vi "CPP-5168-PressureAnalysis.vi"() -> (5 "Plug in titles":string[](array[string]), 7 "Plug in values":string[](array[string]))   [LabVIEW 2011]
uses:
  Globals/Plug_in_data_global.vi
  Globals/Meas_global.vi
panel:
  out "ZeroedCompensatedCalibratedData":dbl[][](array[numeric])
  out "ChannelNames":string[](array[string])
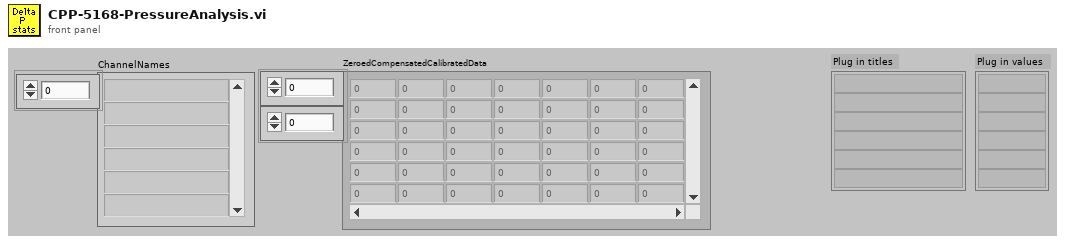
[diagram p1: front panel]
types:
  T1 = typedef "Analysis_info_cluster.ctl" = cluster{"Colour":u32, "Inst type":T2, "Inst name":string, "Symbol":string, "Code name":string, "Extra Info":string, "Inst Array":T3, "Index":i32, "Voltage Index":i32, "Extra Titles":string[], "Extra Values":string[]}
  T2 = typedef "Inst_type.ctl" = enum16{"Propeller anemometer", "Raw voltage", "Pressure Transducer", "Pitot-static tube", "Preston tube", "Hot wire", "Cross wire 1", "Cross wire 2", "Generic Linear", "Generic Polynomial", "Generic BackPoly", "Fast FID", "Thermocouple", "Cold wire", "Pulsed Wire", "LDA Vel", "LDA Tran time", "LDA Arr time"}
  T3 = typedef "Instrument_Array.ctl" = enum16{"PWA", "LDA", "Analogue"}
  T4 = typedef "WindowDescriptor.ctl" = cluster{"WindowName":string, "SurroundingTaps":string[], "TapWeights":dbl[], "OpenAreaFraction":dbl}
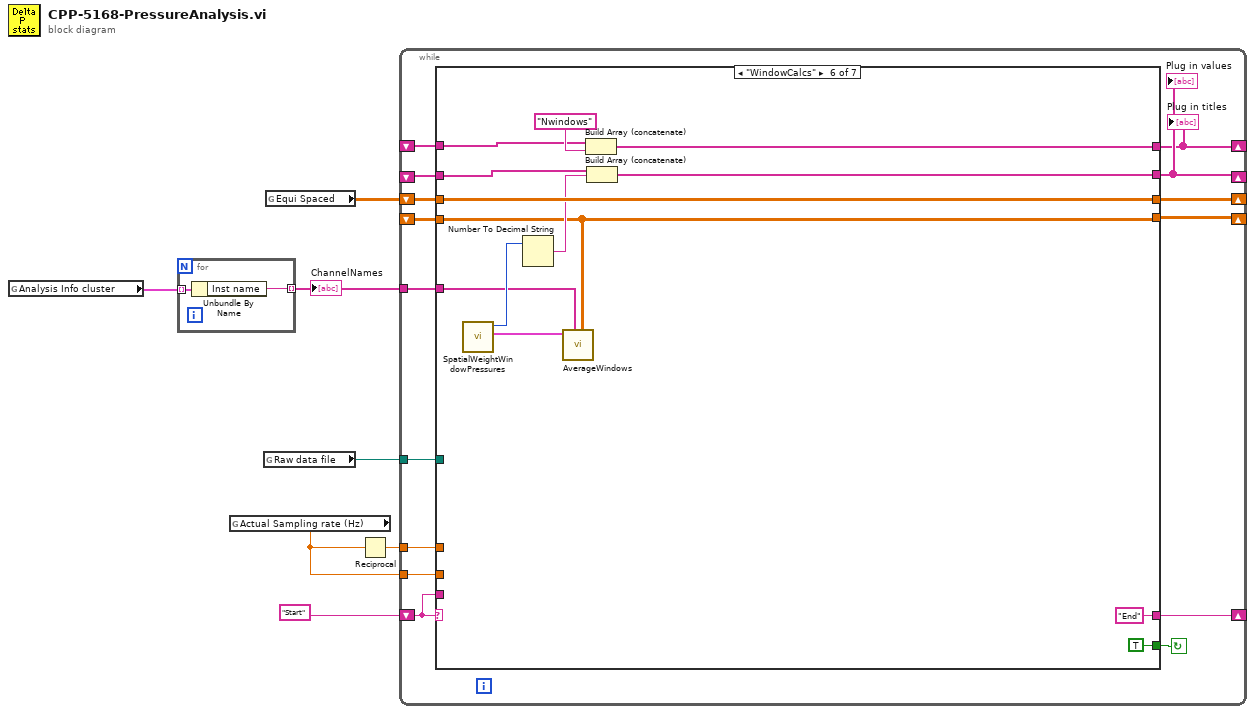
[diagram p0: block diagram]
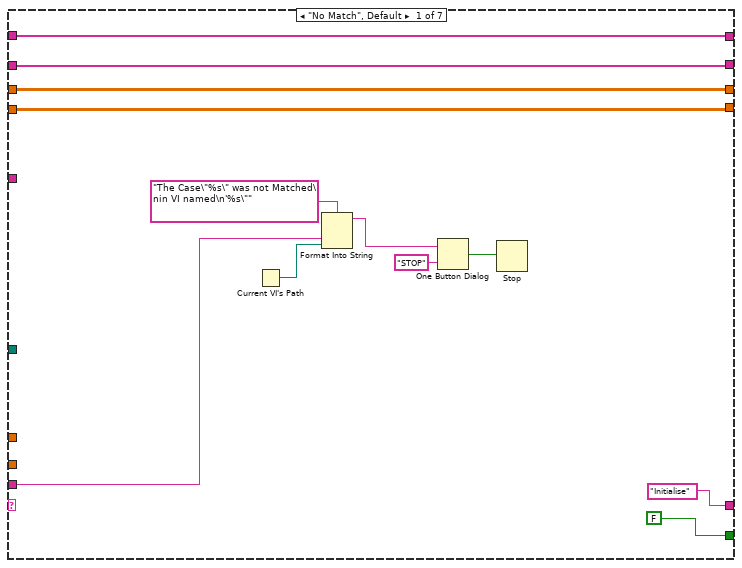
[diagram p2: hidden frame]
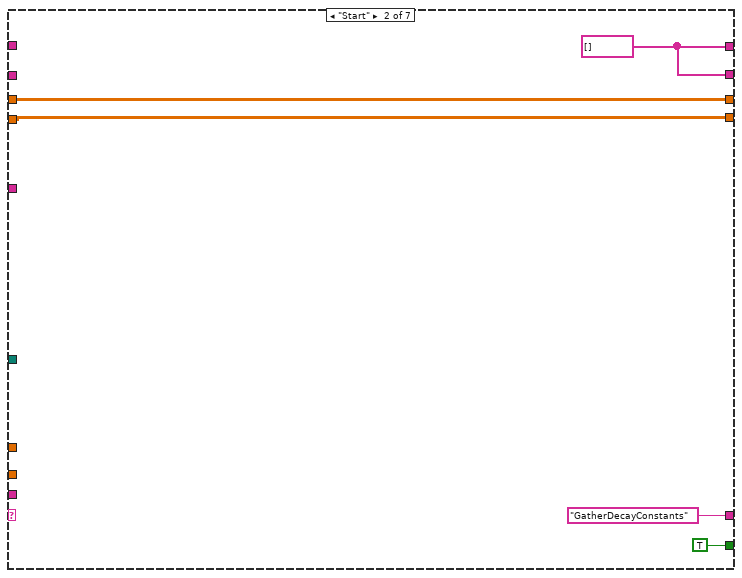
[diagram p3: hidden frame]
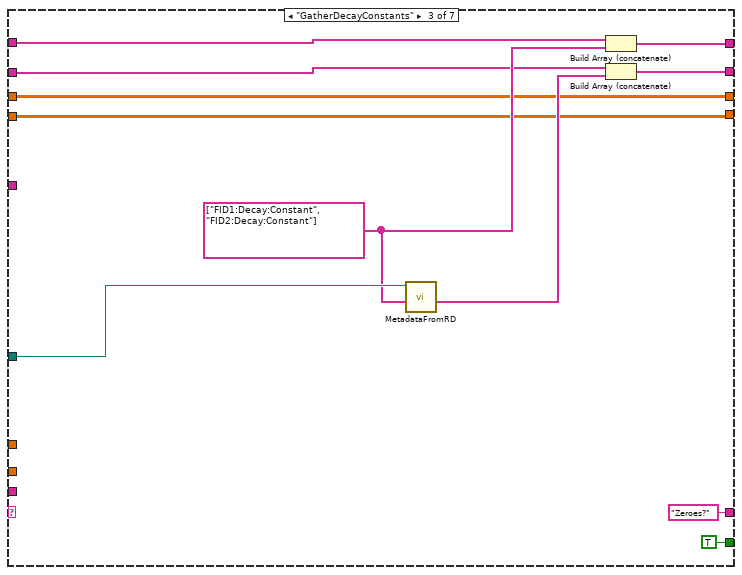
[diagram p4: hidden frame]
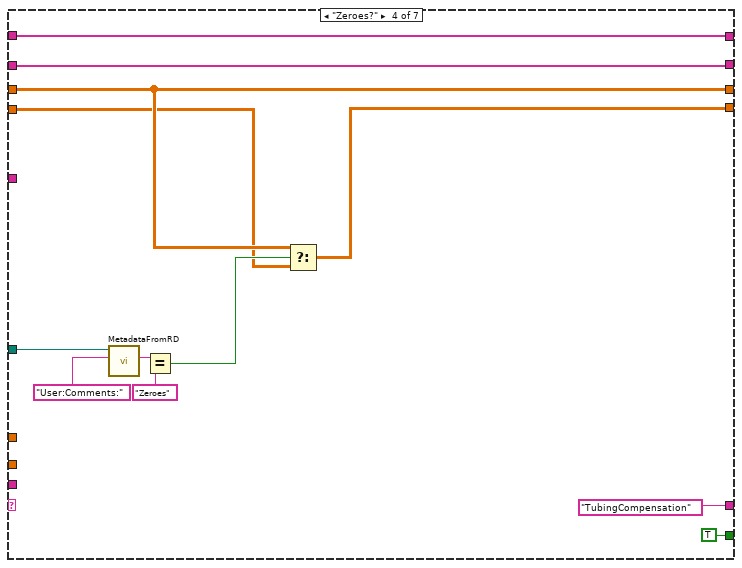
[diagram p5: hidden frame]
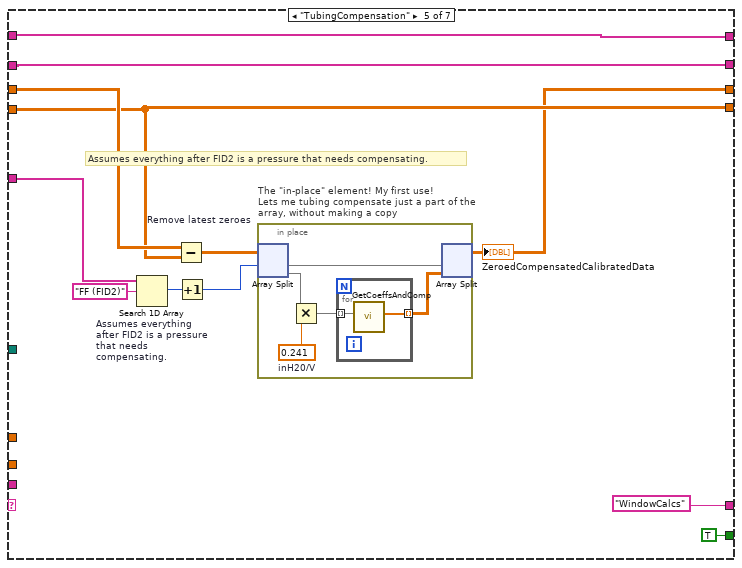
[diagram p6: hidden frame]
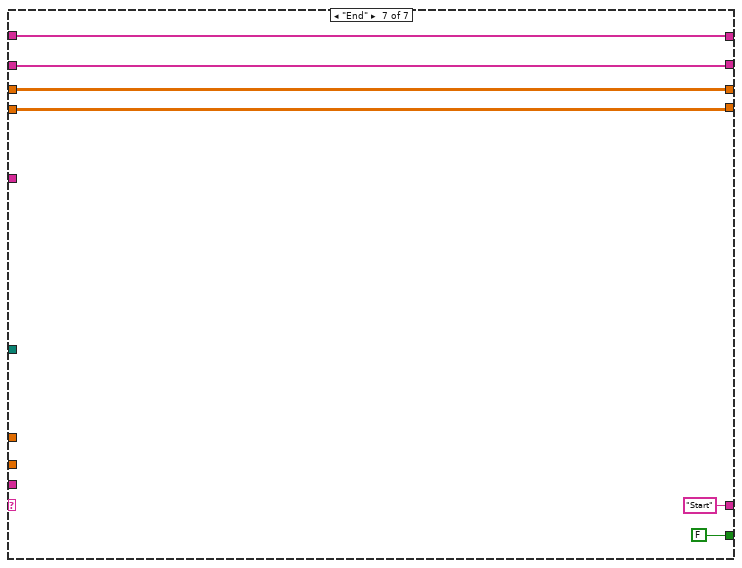
[diagram p7: hidden frame]
diagram:
  n1 = global read "Meas_global.vi" "Analysis Info cluster"() -> (w3:T1[])
  n2 = for {
    tunnel: w3 -> [w9] mode=indexing
    tunnel: [w8] -> w2 mode=indexing
    n3 = Unbundle By Name(w9) -> ("Inst name"=w8:string)
  }
  "ChannelNames" <- w2
  n4 = global read "Meas_global.vi" "Actual Sampling rate (Hz)"() -> (w6:dbl)
  n5 = global read "Meas_global.vi" "Raw data file"() -> (w1:path)
  n6 = global read "Plug_in_data_global.vi" "Equi Spaced"() -> (w4:dbl[][])
  n7 = Reciprocal(x=w6) -> (1/x=w5:dbl)
  n8 = while {
    shift-left: "Start" -> [w22]
    shift-right: [w23] -> _
    tunnel: w6 -> [w21]
    tunnel: w5 -> [w20]
    tunnel: w2 -> [w18]
    tunnel: w1 -> [w17]
    shift-right: [w11] -> _
    shift-left: _ -> [w16]
    shift-right: [w12] -> _
    shift-left: _ -> [w15]
    shift-right: [w14] -> _
    shift-left: _ -> [w13]
    shift-right: [w10] -> _
    shift-left: w4 -> [w19]
    stop <- w24 continue-if-true
    n9 = case shown="\"WindowCalcs\"" w22 {
      tunnel: [FALSE TRUE ("Processing last block?") TRUE ("Processing last block?") TRUE ("Processing last block?") TRUE ("Processing last block?") TRUE ("Processing last block?") FALSE ("Processing last block?")] -> w24
      tunnel: ["Initialise" "GatherDecayConstants" "Zeroes?" ("f") "TubingCompensation" ("f") "WindowCalcs" ("f") "End" ("f") "Start" ("f")] -> w23
      tunnel: w22 -> [w31 _ _ _ _ _ _]
      tunnel: w21 -> [_ _ _ _ _ _ _]
      tunnel: w20 -> [_ _ _ _ _ _ _]
      tunnel: w19 -> [w25 w37 w42 w55 w70 w96 w97]
      tunnel: w18 -> [_ _ _ _ w68 w87 _]
      tunnel: w17 -> [_ _ w50 w64 _ _ _]
      tunnel: w16 -> [w28 _ w47 w62 w66 w90 w100]
      tunnel: [w28 w39 w48 w62 w66 w91 w100] -> w11
      tunnel: [w27 w39 w45 w61 w65 w88 w99] -> w12
      tunnel: w15 -> [w27 _ w44 w61 w65 w89 w99]
      tunnel: [w26 w38 w43 w54 w69 w86 w98] -> w14
      tunnel: w13 -> [w26 w38 w43 w53 w69 w86 w98]
      tunnel: [w25 w37 w42 w55 w67 w96 w97] -> w10
      frame "No Match", Default {
        n10 = Current VI's Path() -> (path=w30:path)
        n11 = Format Into String(format string="The Case\"%s\" was not Matched\nin VI named\n'%s\"" ("Format String"), w31, w30) -> (resulting string=w34:string)  [unwired: 2 in, 1 out]
        n12 = One Button Dialog(message=w34, button name ("OK")="STOP") -> (true=w32:bool)
        n13 = Stop(stop? (T)=w32) -> ()
      }
      frame "Start" {
        w39 = string[] []
      }
      frame "GatherDecayConstants" {
        w49 = string[] ["FID1:Decay:Constant", "FID2:Decay:Constant"] ("Plug in titles")
        n14 = call "MetadataFromRD.vi"("ChannelNames"=w49, "Raw data file"=w50) -> ("ValueStrings"=w46:string[])  [unwired: 8 in, 1 out]
        n15 = Build Array (concatenate)(w47, w49) -> (w48:string[])
        n16 = Build Array (concatenate)(w44, w46) -> (w45:string[])
      }
      frame "Zeroes?" {
        n17 = call "MetadataFromRD.vi"("ChannelName"="User:Comments:", "Raw data file"=w64) -> ("ValueString"=w58:string)  [unwired: 8 in, 1 out]
        n18 = Equal?(x=w58, y="Zeroes") -> (x = y?=w56:bool)
        n19 = Select(t=w55, s=w56, f=w53) -> (s? t:f=w54:dbl[][])
      }
      frame "TubingCompensation" {
        # "Assumes everything after FID2 is a pressure that needs compensating."
        n20 = Search 1D Array "Assumes everything after FID2 is a pressure that needs compensating."(1D array=w68, element="FF (FID2)") -> (index of element=w73:i32)  [unwired: 1 in]
        n21 = Subtract "Remove latest zeroes"(x=w70, y=w69) -> (x-y=w71:dbl[][])
        n22 = Increment(x=w73) -> (x+1=w72:i32)
        n23 = in-place "The \"in-place\" element! My first use!\nLets me tubing compensate just a part of the array, without making a copy" {
          w77 = 0.241  # inH20/V
          n24 = in-place-split #1(w71, w72) -> (w81:dbl[][], w80:dbl[][])
          n25 = Multiply(x=w80, y=w77) -> (x*y=w78:dbl[][])
          n26 = for {
            tunnel: w78 -> [w83] mode=indexing
            tunnel: [w82] -> w79 mode=indexing
            n27 = call "GetCoeffsAndComp.vi"("mutedData"=w83) -> ("boostedData"=w82:dbl[])  [unwired: 10 in]
          }
          n28 = in-place-split #1(w81, w79) -> (w67:dbl[][])  [unwired: 1 out]
        }
        "ZeroedCompensatedCalibratedData" <- w67
      }
      frame "WindowCalcs" {
        n29 = call "SpatialWeightWindowPressures.vi"() -> ("WindowAveragingInformation"=w92:T4[], "nOpen"=w95:i32)  [unwired: 10 in]
        n30 = Number To Decimal String(number=w95) -> (decimal integer string=w94:string)  [unwired: 1 in]
        n31 = call "AverageWindows.vi"("ZeroedCompensatedCalibratedData"=w86, "ChannelNames"=w87, "WindowAveragingInformation"=w92) -> ()  [unwired: 5 in, 2 out]
        n32 = Build Array (concatenate)(w90, "Nwindows") -> (w91:string[])
        n33 = Build Array (concatenate)(w89, w94) -> (w88:string[])
      }
      frame "End" {
      }
    }
    "Plug in values" <- w12
    "Plug in titles" <- w11
  }
